vi "TestFileDaloge.vi"() -> (2 "字符串":string, 3 "选择字符串":string)   [LabVIEW 2018]
panel:
  out "exit":bool
  in  "Bar":bool
  out "All Files in Dir":path[](array[path]) caption="目录中的所有文件"
  out "文件名":string[](array[string])
  in  "取消":bool
  in  "确定":bool
  in  "文件列表":i32(listbox)
  # "测试文件对话框"
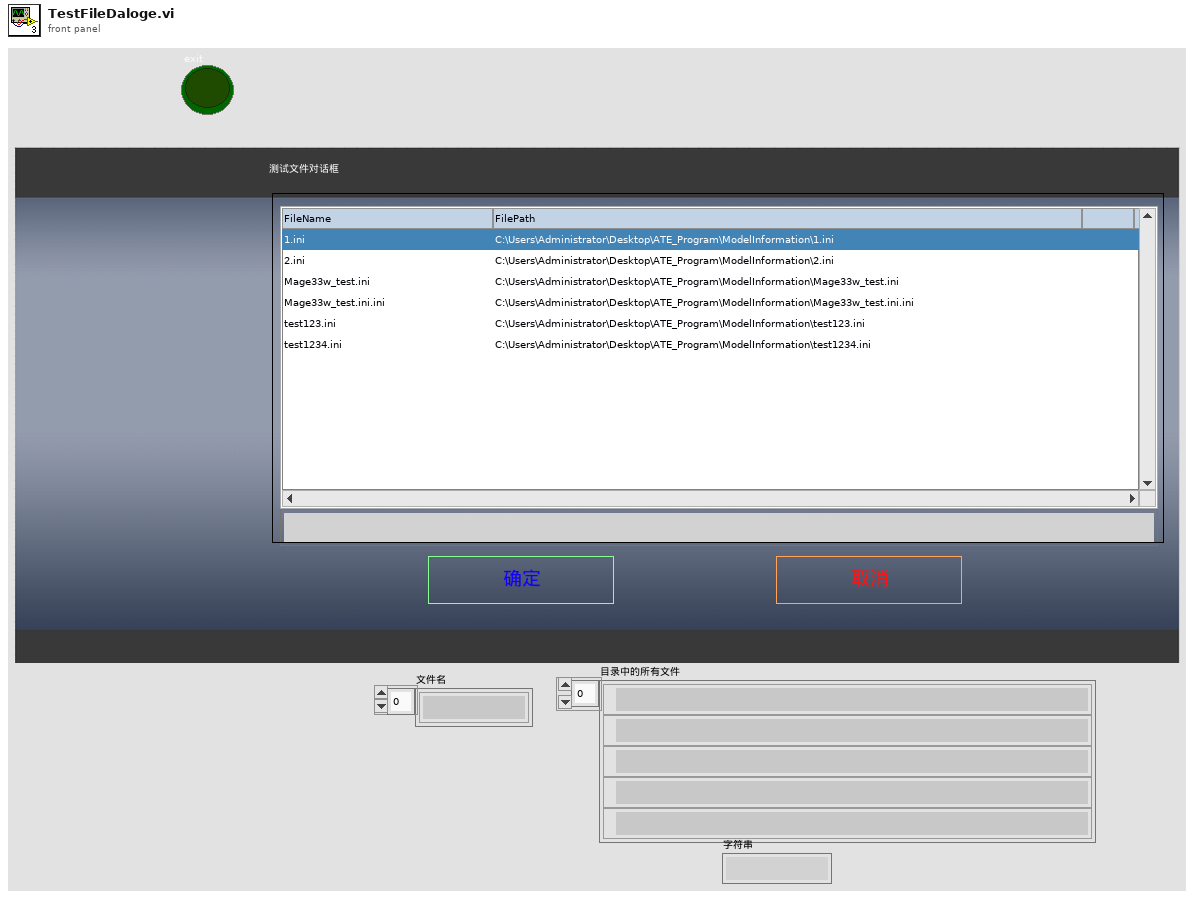
[diagram p1: front panel]
types:
  T1 = typedef "Window Refnum.ctl" = refnum<k1>
  T2 = typedef "Window Rectangle.ctl" = cluster{"left":i16, "top":i16, "right":i16, "bottom":i16}
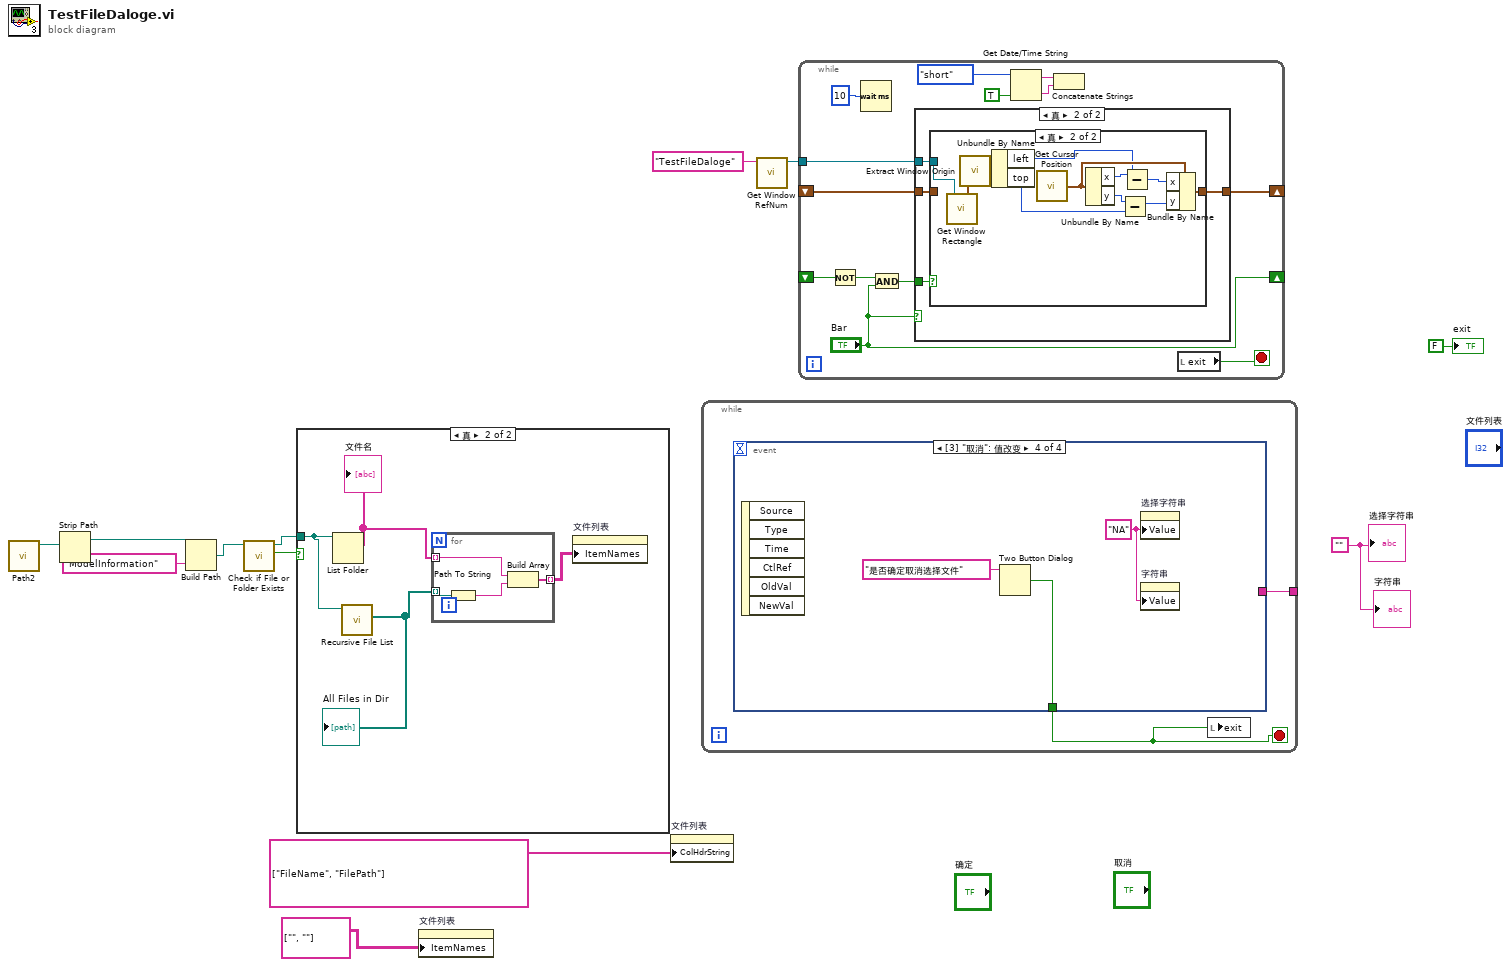
[diagram p0: block diagram]
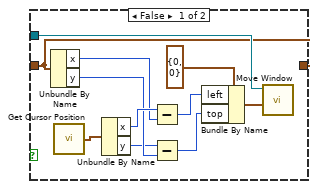
[diagram p3: hidden frame]
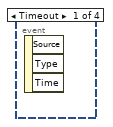
[diagram p5: hidden frame]
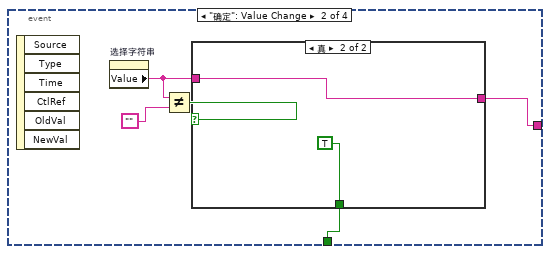
[diagram p6: hidden frame]
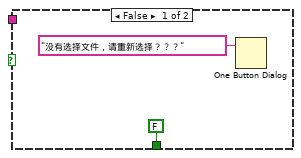
[diagram p7: hidden frame]
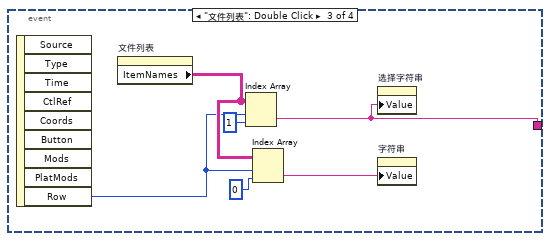
[diagram p8: hidden frame]
diagram:
  w4 = ""
  n1 = call "Path2.vi"() -> ("拆分的路径"=w12:path)  [unwired: 10 in, 1 out]
  n2 = Strip Path(path=w12) -> (stripped path=w11:path)  [unwired: 1 out]
  n3 = Build Path(base path=w11, name or relative path="ModelInformation" ("名称或相对路径")) -> (appended path=w9:path)
  n4 = call <vilib>:"Check if File or Folder Exists.vi"("path"=w9) -> ("file or folder exists?"=w8:bool, "dup path"=w7:path)  [unwired: 8 in, 1 out]
  n5 = case shown="真" w8 {
    tunnel: w7 -> [_ w16]
    frame False {
    }
    frame True {
      n6 = List Folder(path=w16) -> (filenames=w14:string[])  [unwired: 3 in, 3 out]
      "文件名" <- w14
      n7 = call <vilib>:"Recursive File List.vi"("Folder Path"=w16) -> ("All Files in Dir"=w15:path[])  [unwired: 6 in, 4 out]
      "All Files in Dir" <- w15
      n8 = for {
        tunnel: w14 -> [w19] mode=indexing
        tunnel: w15 -> [w20] mode=indexing
        tunnel: [w17] -> w13 mode=indexing
        n9 = Path To String(path=w20) -> (string=w18:string)
        n10 = Build Array(w19, w18) -> (w17:string[])
      }
      n11 = property on="文件列表" class="MCListbox (严格)"("ItemNames"=w13) -> ()  [unwired: 2 in, 2 out]
    }
  }
  n12 = property on="文件列表" class="MCListbox (严格)"("ItemNames"=string[][] [["", ""]] ("列首字符串[]")) -> ()  [unwired: 2 in, 2 out]
  n13 = property on="文件列表" class="MCListbox (严格)"("ColHdrString"=string[] ["FileName", "FilePath"] ("列首字符串[]")) -> ()  [unwired: 2 in, 2 out]
  n14 = while {
    tunnel: [w22] -> _
    stop <- w21 stop-if-true
    n15 = event shown="[3] \"取消\": 值改变" {
      selector: _ -> [_ _ _ _]
      dyn-events: _ -> [_ _ _ _]
      timeout: _ -> [_ _ _ _]
      tunnel: [_ w23 _ w40] -> w21
      tunnel: [_ w25 w36 _] -> w22
      event Timeout {
        n16 = event-data() -> ()  [unwired: 1 in, 3 out]
      }
      event "确定": Value Change {
        n17 = event-data() -> ()  [unwired: 1 in, 6 out]
        n18 = property on="选择字符串" class="Str"() -> ("Value"=w24:string)  [unwired: 2 in, 2 out]
        n19 = Not Equal?(x=w24, y="") -> (x != y?=w26:bool)
        n20 = case shown="真" w26 {
          tunnel: [_ w31] -> w25
          tunnel: w24 -> [_ w31]
          tunnel: [FALSE TRUE] -> w23
          frame False {
            n21 = One Button Dialog(message="没有选择文件，请重新选择？？？" ("消息")) -> ()  [unwired: 1 in, 1 out]
          }
          frame True {
          }
        }
      }
      event "文件列表": Double Click {
        n22 = event-data() -> ("Row"=w33:i32)  [unwired: 1 in, 8 out]
        n23 = property on="文件列表" class="MCListbox (严格)"() -> ("ItemNames"=w35:string[][])  [unwired: 2 in, 2 out]
        n24 = Index Array(array=w35, index (row)=w33, index (col)=1 ("禁用的索引 (列)")) -> (element=w36:string)
        n25 = Index Array(array=w35, index (row)=w33, index (col)=0 ("禁用的索引 (列)")) -> (element=w32:string)
        n26 = property on="选择字符串" class="Str"("Value"=w36) -> ()  [unwired: 2 in, 2 out]
        n27 = property on="字符串" class="Str"("Value"=w32) -> ()  [unwired: 2 in, 2 out]
      }
      event "取消": Value Change {
        w38 = "NA" ("选择字符串")
        n28 = event-data() -> ()  [unwired: 1 in, 6 out]
        n29 = Two Button Dialog(message="是否确定取消选择文件" ("消息")) -> (T button?=w40:bool)  [unwired: 2 in]
        n30 = property on="选择字符串" class="Str"("Value"=w38) -> ()  [unwired: 2 in, 2 out]
        n31 = property on="字符串" class="Str"("Value"=w38) -> ()  [unwired: 2 in, 2 out]
      }
    }
    n32 = local write "exit"(w21) -> ()
  }
  n33 = call "Get Window RefNum.vi"("window name (\"\")"="TestFileDaloge" ("window name (\"\")")) -> ("window refnum (NaWR)"=w3:T1)  [unwired: 1 in, 7 out]
  n34 = while {
    shift-left: _ -> [w47]
    shift-right: [w48] -> _
    shift-left: _ -> [w51]
    shift-right: ["Bar"] -> _
    tunnel: w3 -> [w52]
    stop <- w41 stop-if-true
    n35 = Not(x=w51) -> (.not. x?=w50:bool)
    n36 = Wait (ms)(milliseconds to wait=u32 10) -> ()  [unwired: 1 out]
    n37 = And(x=w50, y="Bar") -> (x .and. y?=w46:bool)
    n38 = case shown="真" "Bar" {
      tunnel: w52 -> [_ w58]
      tunnel: [w54 w57] -> w48
      tunnel: w47 -> [w54 w55]
      tunnel: w46 -> [_ w56]
      frame False {
      }
      frame True {
        n39 = case shown="真" w56 {
          tunnel: w58 -> [w64 w80]
          tunnel: [w59 w70] -> w57
          tunnel: w55 -> [w59 _]
          frame False {
            n40 = Unbundle By Name(w59) -> ("x"=w67:i16, "y"=w66:i16)
            n41 = call "Get Cursor Position.vi"() -> ("cursor position"=w69:cluster{"x":i16, "y":i16})
            n42 = Unbundle By Name(w69) -> ("x"=w68:i16, "y"=w65:i16)
            n43 = Subtract(x=w68, y=w67) -> (x-y=w61:i16)
            n44 = Subtract(x=w65, y=w66) -> (x-y=w62:i16)
            n45 = Bundle By Name(cluster=cluster{"left":i16, "top":i16} {"left"=0, "top"=0} ("new position (0,0)"), "left"=w61, "top"=w62) -> (w60:cluster{"left":i16, "top":i16})
            n46 = call "Move Window.vi"("new position (0,0)"=w60, "window refnum (NaWR)"=w64) -> ()  [unwired: 2 in, 4 out]
          }
          frame True {
            n47 = call "Get Window Rectangle.vi"("window refnum (NaWR)"=w80) -> ("window rect"=w79:T2)  [unwired: 1 in, 5 out]
            n48 = call "Extract Window Origin.vi"("window rect"=w79) -> ("window origin"=w78:cluster{"left":i16, "top":i16})  [unwired: 1 out]
            n49 = Unbundle By Name(w78) -> ("left"=w75:i16, "top"=w74:i16)
            n50 = call "Get Cursor Position.vi"() -> ("cursor position"=w77:cluster{"x":i16, "y":i16})
            n51 = Unbundle By Name(w77) -> ("x"=w76:i16, "y"=w73:i16)
            n52 = Subtract(x=w73, y=w74) -> (x-y=w72:i16)
            n53 = Subtract(x=w76, y=w75) -> (x-y=w71:i16)
            n54 = Bundle By Name(cluster=w77, "x"=w71, "y"=w72) -> (w70:cluster{"x":i16, "y":i16})
          }
        }
      }
    }
    n55 = Get Date/Time String(date format (0)=enum16{"short", "long", "abbreviated"}."short" ("日期格式(0)"), want seconds? (F)=TRUE ("需要秒？(F)")) -> (date string=w44:string, time string=w45:string)  [unwired: 1 in]
    n56 = Concatenate Strings(w44, w45) -> ()  [unwired: 1 out]
    n57 = local read "exit"() -> (w41:bool)
  }
  "选择字符串" <- w4
  "字符串" <- w4
  "exit" <- FALSE ("exit")
